vi "Apply cool-down delay.vi"(8 "error in (no error)":errorcluster, 11 "Logging queue element in":T1 {"Frame Size" items=["100X100"=100, "128X128"=128, "200X200"=200, "256X256"=256, "512X512"=512, "1024x1024"=1024, "2048x2048"=2048]; "Dwell time (us)" format="%#.6g"}) -> (0 "error out":errorcluster)   [LabVIEW 2013]
uses:
  Typedefs/Logging queue element.ctl
  Typedefs/Imaging Protocols enum.ctl
  Typedefs/Frame Size.ctl
  Typedefs/Acquired points count.ctl
  Global Variables/gl_UI Ctrl Refs.vi
panel:
  in  "milliseconds to wait":u32
  in  "(-) Offset (sec)":dbl=0.0013 format="%#_13g"
  # "<--- fine-tuning"
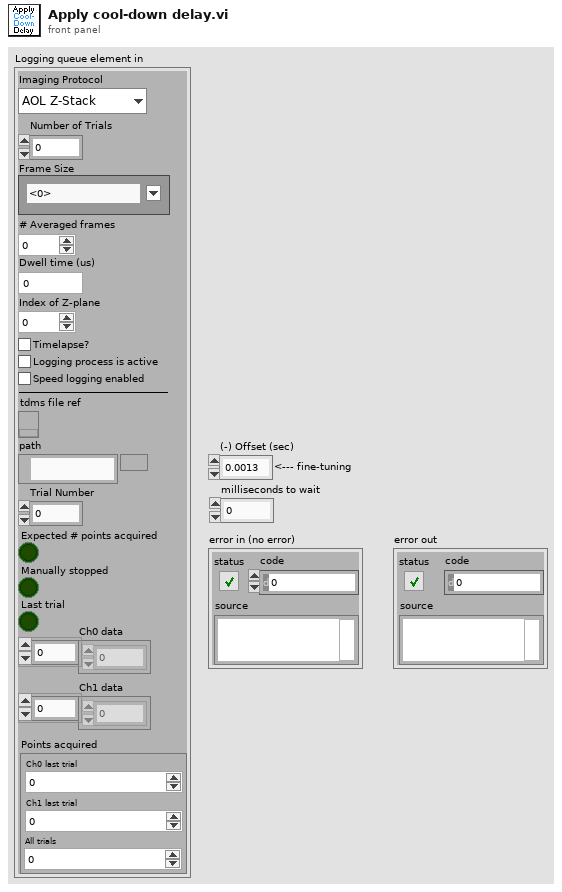
[diagram p1: front panel]
types:
  T1 = typedef "Logging queue element.ctl" = cluster{"Imaging Protocol":T2, "Number of Trials":u16, "Frame Size":T3, "# Averaged frames":u16, "Dwell time (us)":dbl, "Index of Z-plane":i32, "Timelapse?":bool, "Logging process is active":bool, "Speed logging enabled":bool, "tdms file ref":refnum<k34>, "path":path, "Trial Number":i32, "Expected # points acquired":bool, "Manually stopped":bool, "Ch0 data":u32[], "Ch1 data":u32[], "Last trial":bool, "Points acquired":T4}
  T2 = typedef "Imaging Protocols enum.ctl" = enum16{"AOL Z-Stack", "Motor Z Stack", "Functional Acquisition", "Single Plane Acquisition", "Volume Acquisition", "Live Imaging", "Live Plane Imaging", "Live Volume Imaging"}
  T3 = typedef "Frame Size.ctl" = u16
  T4 = typedef "Acquired points count.ctl" = cluster{"Ch0 last trial":u64, "Ch1 last trial":u64, "All trials":u64}
  T5 = typedef "UI ctrl refs cluster.ctl" = cluster{"Top level VI path":path, "Top level VI ref":refnum<vi>, "User menu ref":refnum<k9>, "Sub Panel control":refnum<vi>, "Imaging Param Tab":refnum<vi>, "Occurrence-Start drivers":refnum<k4>, "Occurrence-Speed logging initialised":refnum<k4>, "Occurrence-XYZ stage initialised":refnum<k4>, "Exit button":refnum<vi>, "Status ind":refnum<vi>, "Return to Origin":refnum<vi>, "Speed Logging":refnum<vi>, "Time Lapse":refnum<vi>, "Live Imaging":refnum<vi>, "AOL Z Stack":refnum<vi>, "Motor Z Stack":refnum<vi>, "Funct Acq button":refnum<vi>, "Hard Shutter":refnum<vi>, "Virtual Shutter":refnum<vi>, "Laser Power":refnum<vi>, "AOL Mode":refnum<vi>, "Frame Size":refnum<vi>, "Field of View":refnum<vi>, "Dwell Time":refnum<vi>, "Zoom":refnum<vi>, "AOL Z":refnum<vi>, "Objective":refnum<vi>, "Axis":refnum<vi>, "Paths & Names":refnum<vi>, "Experiment folder path (ind.)":refnum<vi>, "Last State (Ind.)":refnum<vi>, "Laser wavelength ind (nm)":refnum<vi>, "Averages":refnum<vi>, "Angle (degrees)":refnum<vi>, "X centre":refnum<vi>, "Y centre":refnum<vi>, "Plane Mode":refnum<vi>, "# Planes":refnum<vi>, "Z Start":refnum<vi>, "Z Stop":refnum<vi>, "Z Step":refnum<vi>, "PMT 1":refnum<vi>, "PMT 2":refnum<vi>, "Stage XYZ Position":refnum<vi>, "Pockels@Z Start":refnum<vi>, "Pockels@Z Stop":refnum<vi>, "Obtain Z Start":refnum<vi>, "Obtain Z Stop":refnum<vi>, "Live stim.trig.period":refnum<vi>, "Live stim.trig.enable":refnum<vi>, "Funct. Acq. Pockels Modulation":refnum<vi>, "Enable Video Recording":refnum<vi>, "Video Record-Live Imaging":refnum<vi>, "Video Record-Funct acq":refnum<vi>, "AOL Z-stack Chirps Ready (ind)":refnum<vi>, "Center freq ind (nm)":refnum<vi>, "Logging queue (ind)":refnum<vi>, "Back aperture power (ind.)":refnum<vi>, "Power after objective (ind.)":refnum<vi>, "Switch user":refnum<vi>}
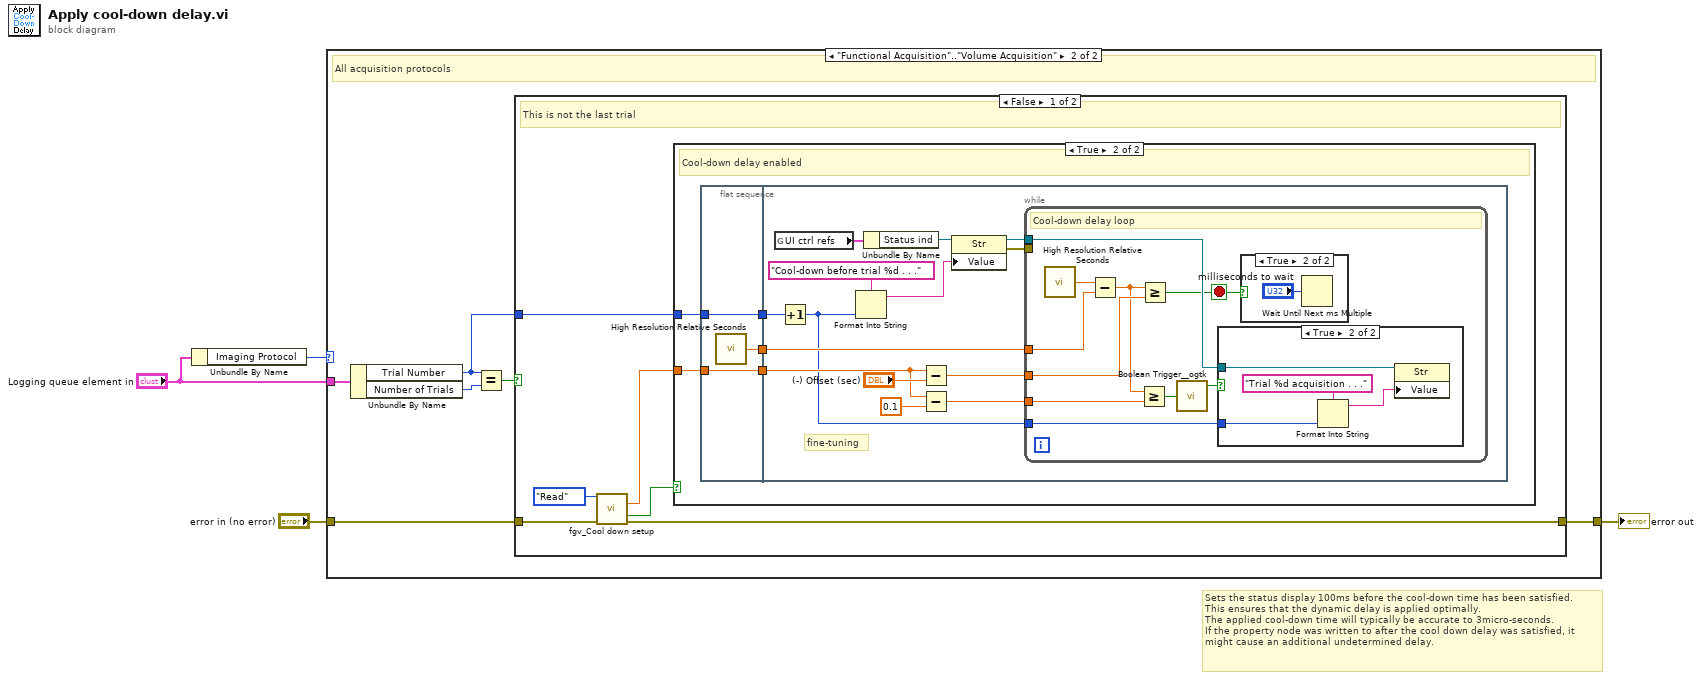
[diagram p0: block diagram]
diagram:
  # "Sets the status display 100ms before the cool-down time has been satisfied.\nThis ensures that the dynamic delay is applied optimally.\nThe applied cool-down time will typically be accurate to 3micro-seconds.\nIf the property node was written to after the cool down delay was satisfied, it might cause an additional undetermined delay."
  n1 = Unbundle By Name("Logging queue element in") -> ("Imaging Protocol"=w2:T2)
  n2 = case shown="\"Functional Acquisition\"..\"Volume Acquisition\"" w2 {
    tunnel: [w5 w11] -> w4
    tunnel: "error in (no error)" -> [w5 w10]
    tunnel: "Logging queue element in" -> [_ w9]
    frame Default {
      # "All other protocols"
    }
    frame "Functional Acquisition".."Volume Acquisition" {
      # "All acquisition protocols"
      n3 = Unbundle By Name(w9) -> ("Trial Number"=w7:i32, "Number of Trials"=w8:u16)
      n4 = Equal?(x=w7, y=w8) -> (x = y?=w6:bool)
      n5 = case shown="False" w6 {
        tunnel: [w17 w55] -> w11
        tunnel: w10 -> [w16 w55]
        tunnel: w7 -> [w12 _]
        frame False {
          # "This is not the last trial"
          n6 = call "fgv_Cool down setup.vi"("Function"=enum16{"Intialize", "Write", "Read", "Clear"}."Read", "error in (no error)"=w16) -> ("Cool-down time (s)"=w13:dbl, "Enable cool-down time"=w14:bool, "error out"=w17:errorcluster)  [unwired: 11 in]
          n7 = case shown="True" w14 {
            tunnel: w13 -> [_ w22]
            tunnel: w12 -> [_ w19]
            frame False {
              # "The status indicator is set by the \"Logging module-status updater.vi\""
              # "Cool-down delay disabled"
            }
            frame True {
              # "Cool-down delay enabled"
              n8 = flat-sequence {
                tunnel: w22 -> [w25]
                tunnel: [w25] -> w21
                tunnel: [w24] -> w20
                tunnel: w19 -> [w23]
                tunnel: [w23] -> w18
                tunnel: w21 -> [w28]
                tunnel: w20 -> [w38]
                tunnel: w18 -> [w27]
                frame #0 {
                  n9 = call <vilib>:"High Resolution Relative Seconds.vi"() -> ("relative seconds"=w24:dbl)
                }
                frame #1 {
                  # "fine-tuning"
                  n10 = global read "gl_UI Ctrl Refs.vi" "UI ctrl refs"() -> (w36:T5)
                  n11 = Increment(x=w27) -> (x+1=w26:i32)
                  n12 = Format Into String(format string="Cool-down before trial %d . . ." ("Acquiring and Logging..."), w26) -> (resulting string=w34:string)  [unwired: 2 in, 1 out]
                  n13 = Unbundle By Name(w36) -> ("Status ind"=w35:refnum<vi>)
                  n14 = Subtract(x=w28, y="(-) Offset (sec)") -> (x-y=w32:dbl)
                  n15 = Subtract(x=w28, y=0.1) -> (x-y=w30:dbl)
                  n16 = property class="Str"(reference=w35, "Value"=w34) -> (reference out=w29:refnum<vi>, error out=w33:errorcluster)  [unwired: 1 in]
                  n17 = while {
                    tunnel: w38 -> [w48]
                    tunnel: w32 -> [w47]
                    tunnel: w33 -> [_]
                    tunnel: w30 -> [w45]
                    tunnel: w29 -> [w42]
                    tunnel: w26 -> [w40]
                    stop <- w41 stop-if-true
                    # "Cool-down delay loop"
                    n18 = call <vilib>:"High Resolution Relative Seconds.vi"() -> ("relative seconds"=w49:dbl)
                    n19 = Subtract(x=w49, y=w48) -> (x-y=w46:dbl)
                    n20 = Greater Or Equal?(x=w46, y=w45) -> (x >= y?=w44:bool)
                    n21 = Greater Or Equal?(x=w46, y=w47) -> (x >= y?=w41:bool)
                    n22 = call "Boolean Trigger__ogtk.vi"("Boolean Input"=w44) -> ("Rising Edge"=w43:bool)  [unwired: 1 in, 1 out]
                    n23 = case shown="True" w43 {
                      tunnel: w42 -> [_ w53]
                      tunnel: w40 -> [_ w50]
                      frame False {
                      }
                      frame True {
                        n24 = Format Into String(format string="Trial %d acquisition . . ." ("Acquiring and Logging..."), w50) -> (resulting string=w51:string)  [unwired: 2 in, 1 out]
                        n25 = property class="Str"(reference=w53, "Value"=w51) -> ()  [unwired: 1 in, 2 out]
                      }
                    }
                    n26 = case shown="True" w41 {
                      frame False {
                      }
                      frame True {
                        n27 = Wait Until Next ms Multiple(millisecond multiple="milliseconds to wait") -> ()  [unwired: 1 out]
                      }
                    }
                  }
                }
              }
            }
          }
        }
        frame True {
          # "Last trial"
        }
      }
    }
  }
  "error out" <- w4
